vi "DigitalRead_Single.vi"(2 "error in":errorcluster, 3 "Channel":refnum<k21>) -> (0 "error out":errorcluster, 1 "data":bool)   [LabVIEW 2011]
uses:
  <vilib>/DAQmx/read.llb/DAQmx Read (Digital Bool 1Line 1Point).vi
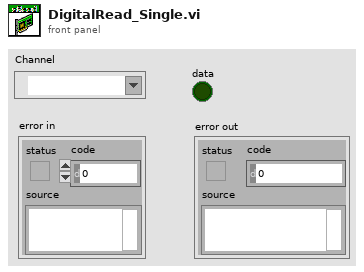
[diagram p1: front panel]
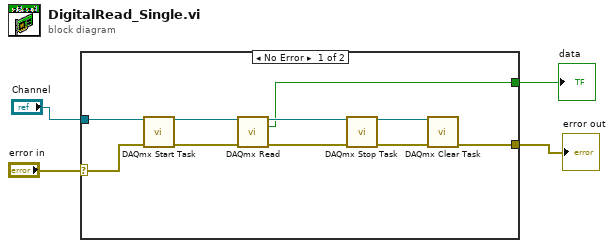
[diagram p0: block diagram]
diagram:
  n1 = case shown="No Error" "error in" {
    selector: "error in" -> [w7 w15]
    tunnel: [w8 w15] -> w1
    tunnel: "Channel" -> [w6 _]
    tunnel: [w5 _] -> w2
    frame No Error {
      n2 = call <vilib>:"DAQmx Start Task.vi"("task/channels in"=w6, "error in"=w7) -> ("task out"=w12:refnum<k21>, "error out"=w14:errorcluster)  [unwired: 12 in]
      n3 = call-poly <vilib>:"DAQmx Read.vi"("task/channels in"=w12, "error in"=w14) -> ("task out"=w11:refnum<k21>, "data"=w5:bool, "error out"=w13:errorcluster)  [unwired: 11 in]
      n4 = call <vilib>:"DAQmx Stop Task.vi"("task/channels in"=w11, "error in"=w13) -> ("task out"=w10:refnum<k21>, "error out"=w9:errorcluster)  [unwired: 12 in]
      n5 = call <vilib>:"DAQmx Clear Task.vi"("task in"=w10, "error in"=w9) -> ("error out"=w8:errorcluster)  [unwired: 13 in]
    }
    frame Error {
    }
  }
  "data" <- w2
  "error out" <- w1
